vi "AppendParamNamesNumbers.vi"   [LabVIEW 2015]
uses:
  GlobalDataNames.vi
  GlobalDataNum.vi
  GlobalDataFileRefnum7.vi
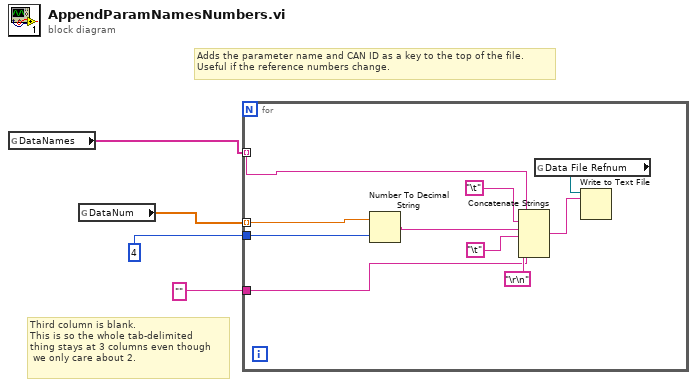
[diagram p0: block diagram]
diagram:
  # "Third column is blank.\nThis is so the whole tab-delimited\nthing stays at 3 columns even though\n we only care about 2."
  # "Adds the parameter name and CAN ID as a key to the top of the file.\nUseful if the reference numbers change."
  n1 = global read "GlobalDataNames.vi" "DataNames"() -> (w2:string[])
  n2 = global read "GlobalDataNum.vi" "DataNum"() -> (w1:dbl[])
  n3 = for {
    tunnel: w1 -> [w8] mode=indexing
    tunnel: 4 -> [w7]
    tunnel: "" -> [w6]
    tunnel: w2 -> [w5] mode=indexing
    n4 = Number To Decimal String(number=w8, width (-)=w7) -> (decimal integer string=w14:string)
    n5 = Concatenate Strings(w5, "\t", w14, "\t", w6, "\r\n") -> (w11:string)
    n6 = global read "GlobalDataFileRefnum7.vi" "Data File Refnum"() -> (w9:refnum<file>)
    n7 = Write to Text File(file (use dialog)=w9, text=w11) -> ()  [unwired: 2 in, 3 out]
  }
